vi "FT_Open_Device.vi"(7 "Flags":u32(ring)=2 items=["FT_OPEN_BY_SERIAL_NUMBER"=1, "FT_OPEN_BY_DESCRIPTION"=2, "FT_OPEN_BY_LOCATION"=4], 8 "error in (no error)":errorcluster, 11 "Device Description":string) -> (0 "error out":errorcluster, 1 "FT_Status":u32(ring) items=["FT_OK", "FT_INVALID_HANDLE", "FT_DEVICE_NOT_FOUND", "FT_DEVICE_NOT_OPENED", "FT_IO_ERROR", "FT_INSUFFICIENT_RESOURCES", "FT_INVALID_PARAMETER", "FT_INVALID_BAUD_RATE", "FT_DEVICE_NOT_OPENED_FOR_ERASE", "FT_DEVICE_NOT_OPENED_FOR_WRITE", "FT_FAILED_TO_WRITE_DEVICE", "FT_EEPROM_READ_FAILED", "FT_EEPROM_WRITE_FAILED", "FT_EEPROM_ERASE_FAILED", "FT_EEPROM_NOT_PRESENT", "FT_EEPROM_NOT_PROGRAMMED", "FT_INVALID_ARGS", "FT_NOT_SUPPORTED", "FT_OTHER_ERROR"], 3 "Handle":u64)   [LabVIEW 2018]
uses:
  FTD2XX.dll
panel:
  in  "device":i32
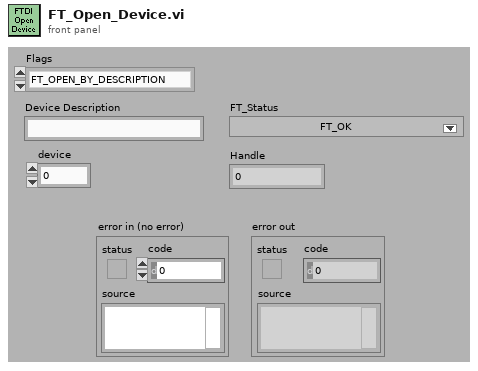
[diagram p1: front panel]
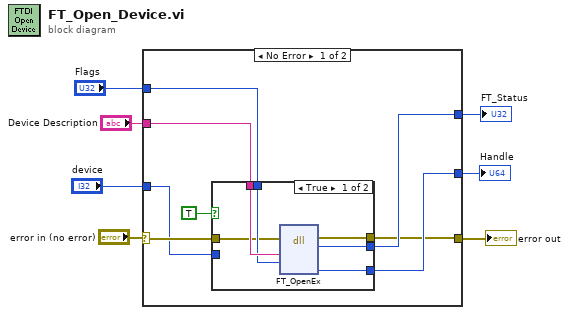
[diagram p0: block diagram]
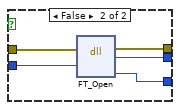
[diagram p2: hidden frame]
diagram:
  n1 = case shown="No Error" "error in (no error)" {
    selector: "error in (no error)" -> [w12 w27]
    tunnel: [w15 _] -> w7
    tunnel: [w14 _] -> w6
    tunnel: "Device Description" -> [w13 _]
    tunnel: [w11 w27] -> w3
    tunnel: "device" -> [w9 _]
    tunnel: "Flags" -> [w8 _]
    frame No Error {
      n2 = case shown="True" TRUE {
        tunnel: [w21 w26] -> w15
        tunnel: [w20 w25] -> w14
        tunnel: w13 -> [w19 _]
        tunnel: w8 -> [w18 _]
        tunnel: w12 -> [w17 w24]
        tunnel: [w16 w23] -> w11
        tunnel: w9 -> [_ w22]
        frame True {
          n3 = dll-call lib="FTD2XX.dll" fn="FT_OpenEx"(error in=w17, "DeviceDescription"=w19, "Flags"=w18) -> (error out=w16:errorcluster, "FT_Status"=w20:u32, "Handle"=w21:u64)  [unwired: 5 in, 1 out]
        }
        frame False {
          n4 = dll-call lib="FTD2XX.dll" fn="FT_Open"(error in=w24, "device"=w22) -> (error out=w23:errorcluster, "FT_Status"=w25:u32, "Handle"=w26:u64)  [unwired: 4 in, 1 out]
        }
      }
    }
    frame Error {
    }
  }
  "Handle" <- w7
  "FT_Status" <- w6
  "error out" <- w3
